vi "AddAttributes.vi"(8 "error in":errorcluster, 9 "OwningElement in":refnum<k20>, 10 "Document in":refnum<k20>, 11 "Attributes":refnum<class "Attribute.lvclass">[](array[class])) -> (0 "error out":errorcluster, 1 "OwningElement out":refnum<k20>, 2 "Document out":refnum<k20>)   [LabVIEW 2021, in "ProligentXMLGenerator.lvlib" / "DOMSupport.lvlib"]
uses:
  DOMSupport.lvlib
  Attribute/Attribute.lvclass
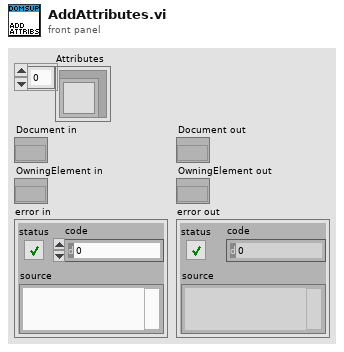
[diagram p1: front panel]
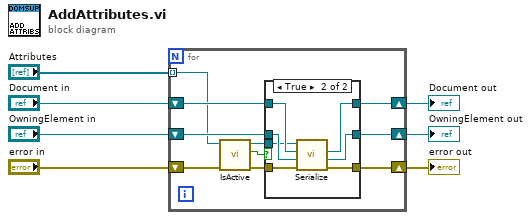
[diagram p0: block diagram]
diagram:
  n1 = for {
    tunnel: "Attributes" -> [w12] mode=indexing
    shift-right: [w9] -> w2
    shift-left: "Document in" -> [w17]
    shift-right: [w8] -> w1
    shift-left: "OwningElement in" -> [w15]
    shift-right: [w10] -> w7
    shift-left: "error in" -> [w11]
    n2 = call "IsActive.vi"("error in"=w11, "Attribute in"=w12) -> ("error out"=w16:errorcluster, "IsActive"=w13:bool, "Attribute out"=w14:refnum<class "Attribute.lvclass">)  [unwired: 7 in]
    n3 = case shown="True" w13 {
      tunnel: w17 -> [w19 w27]
      tunnel: w16 -> [w20 w26]
      tunnel: w15 -> [w18 w25]
      tunnel: [w20 w24] -> w10
      tunnel: w14 -> [_ w23]
      tunnel: [w19 w22] -> w9
      tunnel: [w18 w21] -> w8
      frame False {
      }
      frame True {
        n4 = call "Serialize.vi"("error in"=w26, "OwningElement in"=w25, "Document in"=w27, "Attribute in"=w23) -> ("error out"=w24:errorcluster, "OwningElement out"=w21:refnum<k20>, "Document out"=w22:refnum<k20>)  [unwired: 4 in, 1 out]
      }
    }
  }
  "error out" <- w7
  "Document out" <- w2
  "OwningElement out" <- w1
